vi "Color Change.vi"(2 "Colors":u32[](array[colorbox]), 3 "Configured Inst Input":T1[](array[typedef]) {"Private"."Offset" format="%^_3e"; "Private"."Scale Factors" format="%^_3e"}) -> (0 "Configured Inst dup":T1[](array[typedef]) {"Private"."Offset" format="%^_3e"; "Private"."Scale Factors" format="%^_3e"})   [LabVIEW 2021]
uses:
  Sub Controls/Instrument Properties.ctl
  Sub Controls/Public.ctl
  Sub Controls/Private.ctl
  Sub Controls/Instrument Ref.ctl
  Sub Controls/SystemCheckBox-resize.ctl
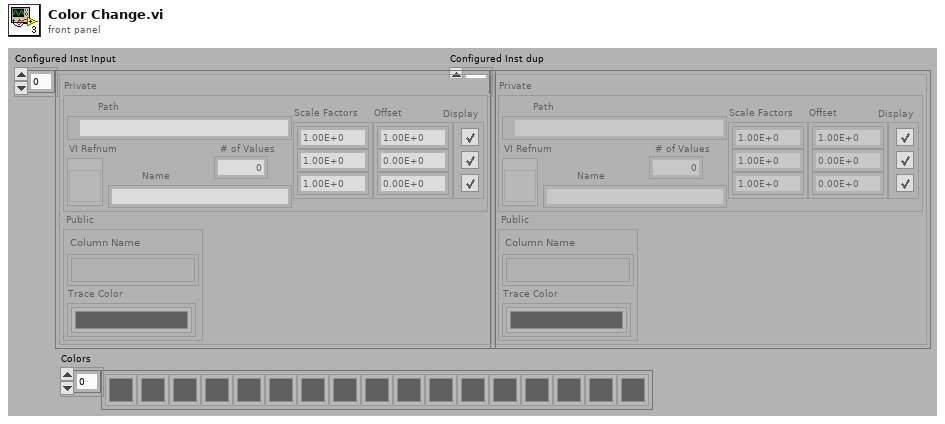
[diagram p1: front panel]
types:
  T1 = typedef "Instrument Properties.ctl" = cluster{"Public":T2, "Private":T3}
  T2 = typedef "Public.ctl" = cluster{"Column Name":string[], "Trace Color":u32[]}
  T3 = typedef "Private.ctl" = cluster{"Path":path, "VI Refnum":T4, "Name":string, "# of Values":i32, "Scale Factors":dbl[], "Display":T5[], "Offset":dbl[]}
  T4 = typedef "Instrument Ref.ctl" = refnum<vi>
  T5 = typedef "SystemCheckBox-resize.ctl" = bool
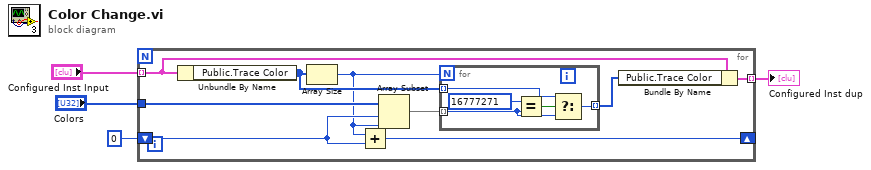
[diagram p0: block diagram]
diagram:
  n1 = for {
    tunnel: "Configured Inst Input" -> [w11] mode=indexing
    shift-right: [w13] -> _
    shift-left: 0 -> [w9]
    tunnel: "Colors" -> [w12]
    tunnel: [w10] -> w4 mode=indexing
    n2 = Unbundle By Name(w11) -> ("Public.Trace Color"=w7:u32[])
    n3 = Array Size(array=w7) -> (size(s)=w6:i32)
    n4 = Add(x=w6, y=w9) -> (x+y=w13:i32)
    n5 = Array Subset(array=w12, index=w9, length=w6) -> (w8:u32[])
    n6 = for {
      N: w6 -> [_]
      tunnel: w8 -> [w15] mode=indexing
      tunnel: w7 -> [w17] mode=indexing
      tunnel: [w14] -> w5 mode=indexing
      n7 = Equal?(x=u32 16777271, y=w15) -> (x = y?=w16:bool)
      n8 = Select(t=w17, s=w16, f=w15) -> (s? t:f=w14:u32)
    }
    n9 = Bundle By Name(cluster=w11, "Public.Trace Color"=w5) -> (w10:T1)
  }
  "Configured Inst dup" <- w4
